vi "FLAT SEQUENCE OF TRAFFIC LIGHTS.vi"() -> ()   [LabVIEW 2018]
panel:
  out "YELLOW":bool
  out "GREEN":bool
  out "RED":bool
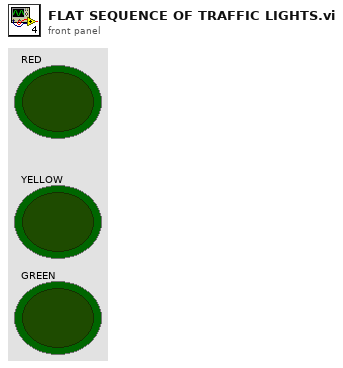
[diagram p1: front panel]
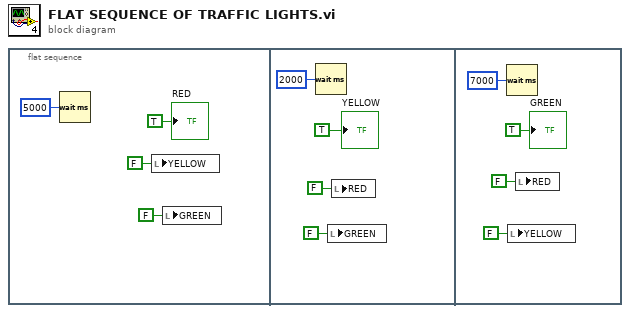
[diagram p0: block diagram]
diagram:
  n1 = flat-sequence {
    frame #0 {
      n2 = Wait (ms)(milliseconds to wait=u32 5000) -> ()  [unwired: 1 out]
      n3 = local write "YELLOW"(FALSE ("YELLOW")) -> ()
      n4 = local write "GREEN"(FALSE ("GREEN")) -> ()
      "RED" <- TRUE ("RED")
    }
    frame #1 {
      n5 = Wait (ms)(milliseconds to wait=u32 2000) -> ()  [unwired: 1 out]
      n6 = local write "GREEN"(FALSE ("GREEN")) -> ()
      n7 = local write "RED"(FALSE ("RED")) -> ()
      "YELLOW" <- TRUE ("YELLOW")
    }
    frame #2 {
      n8 = Wait (ms)(milliseconds to wait=u32 7000) -> ()  [unwired: 1 out]
      n9 = local write "YELLOW"(FALSE ("YELLOW")) -> ()
      n10 = local write "RED"(FALSE ("RED")) -> ()
      "GREEN" <- TRUE ("GREEN")
    }
  }
